vi "EventLoop.vi"() -> ()   [LabVIEW 2020]
panel:
  in  "STOP":bool
  in  "Button 2":bool
  in  "Button 1":bool
  out "error out":errorcluster
  in  "error in":errorcluster
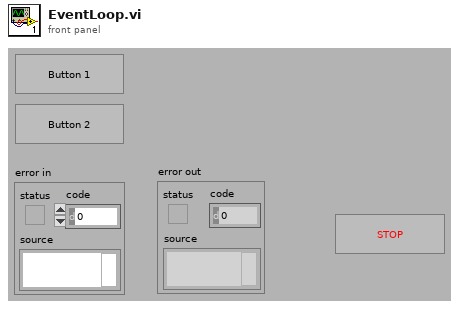
[diagram p1: front panel]
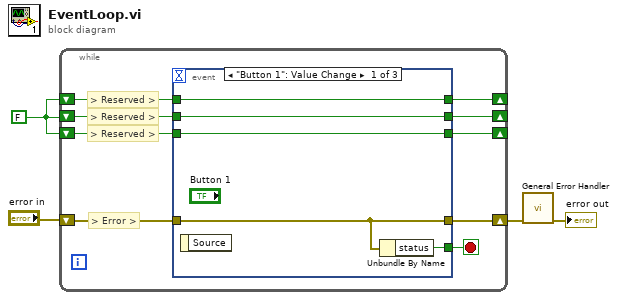
[diagram p0: block diagram]
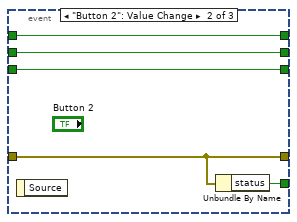
[diagram p2: hidden frame]
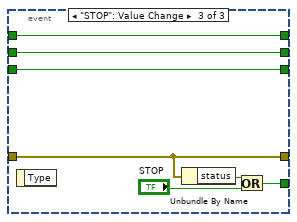
[diagram p3: hidden frame]
diagram:
  w2 = FALSE
  n1 = while {
    shift-right: [w11] -> w4
    shift-left: "error in" -> [w12]
    shift-right: [w9] -> _
    shift-left: w2 -> [w10]
    shift-right: [w7] -> _
    shift-left: w2 -> [w8]
    shift-right: [w5] -> _
    shift-left: w2 -> [w6]
    stop <- w13 stop-if-true
    # "> Reserved >"
    # "> Reserved >"
    # "> Error >"
    # "> Reserved >"
    n2 = event shown="[0] \"Button 1\": Value Change" {
      selector: _ -> [_ _ _]
      dyn-events: _ -> [_ _ _]
      timeout: _ -> [_ _ _]
      tunnel: [w17 w22 w29] -> w13
      tunnel: w12 -> [w18 w23 w25]
      tunnel: [w18 w23 w25] -> w11
      tunnel: w10 -> [w16 w21 w28]
      tunnel: [w16 w21 w28] -> w9
      tunnel: w8 -> [w15 w20 w27]
      tunnel: [w15 w20 w27] -> w7
      tunnel: w6 -> [w14 w19 w26]
      tunnel: [w14 w19 w26] -> w5
      event "Button 1": Value Change {
        n3 = event-data() -> ()  [unwired: 1 in, 1 out]
        n4 = Unbundle By Name(w18) -> ("status"=w17:bool)
      }
      event "Button 2": Value Change {
        n5 = event-data() -> ()  [unwired: 1 in, 1 out]
        n6 = Unbundle By Name(w23) -> ("status"=w22:bool)
      }
      event "STOP": Value Change {
        n7 = event-data() -> ()  [unwired: 1 in, 1 out]
        n8 = Unbundle By Name(w25) -> ("status"=w30:bool)
        n9 = Or(x=w30, y="STOP") -> (x .or. y?=w29:bool)
      }
    }
  }
  n10 = call <vilib>:"General Error Handler.vi"("error in (no error)"=w4) -> ("error out"=→"error out":errorcluster)  [unwired: 10 in, 4 out]
